vi "initialise__.vi"(8 "error in (no error)":errorcluster, 11 "GenericTrajectory in":refnum<class "TrajectoryDL110413StraightLine.lvclass">) -> (0 "error out":errorcluster, 3 "GenericTrajectory out":refnum<class "TrajectoryDL110413StraightLine.lvclass">)   [LabVIEW 2010]
uses:
  <vilib>/Analysis/NI_AALBase.lvlib
  <vilib>/Analysis/1siggen.llb/Ramp Pattern by Samples.vi
  TrajectoryDL110413StraightLine.lvclass
  common/enumerations/functional_global_action_enum.ctl
  common/enumerations/x_y_z_enumeration.ctl
  common/classes/ImageCollection/ImageCollection/ImageCollection.lvclass
  common/classes/Image/Image/Image.lvclass
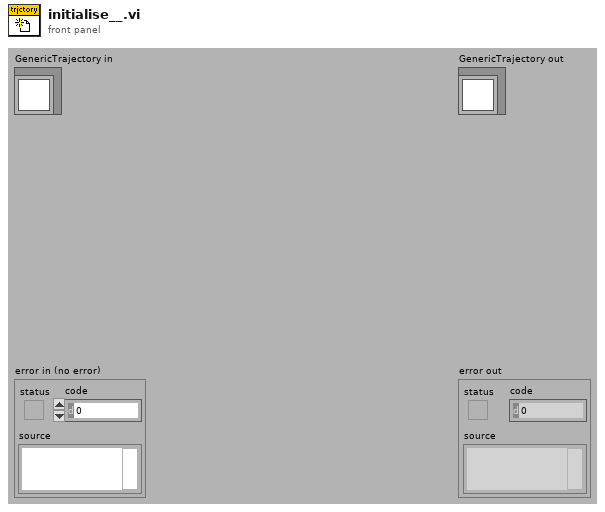
[diagram p1: front panel]
types:
  T1 = typedef "x_y_z_enumeration.ctl" = enum16{"x", "y", "z"}
  T2 = typedef "functional_global_action_enum.ctl" = enum16{"get", "set", "reset"}
  T3 = cluster{"[0]":void, "[1]":void, "[2]":void, "[3]":void}
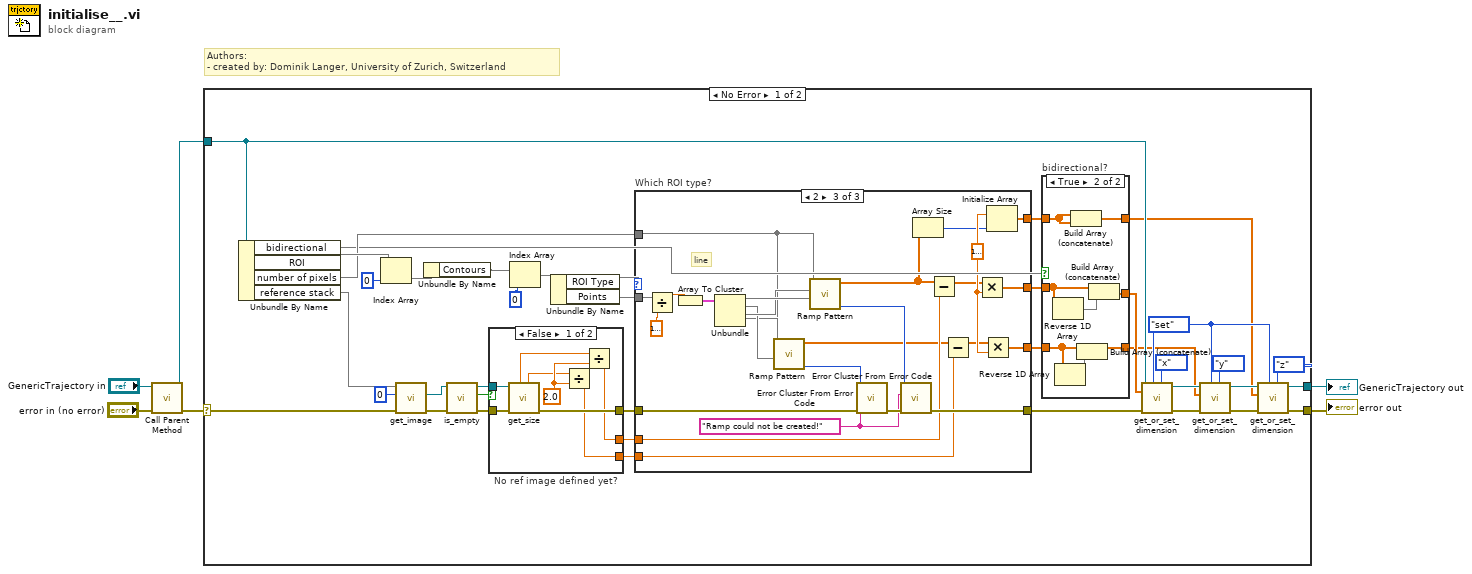
[diagram p0: block diagram]
diagram:
  # "Authors: \n- created by: Dominik Langer, University of Zurich, Switzerland"
  n1 = call-parent "Call Parent Method"("error in (no error)"="error in (no error)", "GenericTrajectory in"="GenericTrajectory in") -> ("error out"=w4:errorcluster, "GenericTrajectory out"=w3:refnum<class "TrajectoryDL110413StraightLine.lvclass">)  [unwired: 8 in]
  n2 = case shown="No Error" w4 {
    selector: w4 -> [w22 w94]
    tunnel: w3 -> [w36 w95]
    tunnel: [w29 w95] -> w2
    tunnel: [w27 w94] -> w1
    frame No Error {
      w26 = functional_global_action_enum."set" ("action")
      n3 = Unbundle By Name(w36) -> ("bidirectional"=w9, "ROI"=w45, "number of pixels"=w37, "reference stack"=w24)
      n4 = Index Array(array=w45, index=0) -> (element=w43)
      n5 = call-dynamic "get_image.vi"("error in (no error)"=w22, "index"=0, "ImageCollection in"=w24) -> ("error out"=w18:errorcluster, "Image.lvclass"=w16:refnum<class "Image.lvclass">)  [unwired: 6 in, 1 out]
      n6 = Unbundle By Name(w43) -> ("Contours"=w41)
      n7 = call-dynamic "is_empty.vi"("error in (no error)"=w18, "Image in"=w16) -> ("error out"=w17:errorcluster, "emtpy?"=w14:bool, "Image out"=w15:refnum<class "Image.lvclass">)  [unwired: 7 in]
      n8 = case "No ref image defined yet?" shown="False" w14 {
        tunnel: [w64 w65] -> w21
        tunnel: [w61 _] -> w20
        tunnel: [w59 _] -> w19
        tunnel: w17 -> [w58 w65]
        tunnel: w15 -> [w57 _]
        frame False {
          w63 = 2.0 ("y")
          n9 = call-dynamic "get_size.vi"("error in (no error)"=w58, "Image in"=w57) -> ("error out"=w64:errorcluster, "physical size y"=w60:dbl, "physical size x"=w62:dbl)  [unwired: 2 in, 5 out]
          n10 = Divide(x=w60, y=w63) -> (x/y=w59:dbl)
          n11 = Divide(x=w62, y=w63) -> (x/y=w61:dbl)
        }
        frame True {
        }
      }
      n12 = Index Array(array=w41, index=0) -> (element=w40)
      n13 = Unbundle By Name(w40) -> ("ROI Type"=w39, "Points"=w38)
      n14 = case "Which ROI type?" shown="2" w39 {
        tunnel: w38 -> [_ _ w91]
        tunnel: w37 -> [_ _ w68]
        tunnel: w21 -> [w66 w67 w84]
        tunnel: [w66 w67 w81] -> w34
        tunnel: [_ _ w75] -> w13
        tunnel: [_ _ w80] -> w10
        tunnel: [_ _ w77] -> w8
        tunnel: w20 -> [_ _ w74]
        tunnel: w19 -> [_ _ w71]
        frame Default {
        }
        frame 1 {
          # "single points..."
        }
        frame 2 {
          w76 = "Ramp could not be created!" ("error message (\"\")")
          w79 = dbl[unit] 1e-06 ("y")
          # "line"
          n15 = Divide(x=w91, y=dbl[unit] 1e-06) -> (x/y=w90:dbl)
          n16 = Array To Cluster(array=w90) -> (cluster=w93:T3)
          n17 = Unbundle(w93) -> ("[0]"=w89, "[1]"=w87, "[2]"=w88, "[3]"=w86)
          n18 = call-poly <vilib>:"Ramp Pattern.vi"("start"=w87, "end"=w86, "samples"=w68) -> ("error"=w85:i32, "Ramp Pattern"=w70:dbl[])  [unwired: 7 in]
          n19 = call-poly <vilib>:"Ramp Pattern.vi"("start"=w89, "end"=w88, "samples"=w68) -> ("error"=w83:i32, "Ramp Pattern"=w73:dbl[])  [unwired: 7 in]
          n20 = call <vilib>:"Error Cluster From Error Code.vi"("error in (no error)"=w84, "error message (\"\")"=w76, "error code (0)"=w85) -> ("error out"=w82:errorcluster)  [unwired: 6 in]
          n21 = call <vilib>:"Error Cluster From Error Code.vi"("error in (no error)"=w82, "error message (\"\")"=w76, "error code (0)"=w83) -> ("error out"=w81:errorcluster)  [unwired: 6 in]
          n22 = Array Size(array=w73) -> (size(s)=w78:i32)
          n23 = Subtract(x=w73, y=w74) -> (x-y=w72:dbl[])
          n24 = Subtract(x=w70, y=w71) -> (x-y=w69:dbl[])
          n25 = Multiply(x=w72, y=w79) -> (x*y=w75:dbl[unit][])
          n26 = Multiply(x=w69, y=w79) -> (x*y=w80:dbl[unit][])
          n27 = Initialize Array(w79, w78) -> (w77:dbl[unit][])
        }
      }
      n28 = case "bidirectional?" shown="True" w9 {
        tunnel: w13 -> [w47 w56]
        tunnel: [w47 w54] -> w12
        tunnel: [w48 w52] -> w11
        tunnel: w10 -> [w48 w51]
        tunnel: w8 -> [w46 w50]
        tunnel: [w46 w49] -> w7
        frame False {
        }
        frame True {
          n29 = Reverse 1D Array(array=w56) -> (reversed array=w55:dbl[unit][])
          n30 = Reverse 1D Array(array=w51) -> (reversed array=w53:dbl[unit][])
          n31 = Build Array (concatenate)(w50, w50) -> (w49:dbl[unit][])
          n32 = Build Array (concatenate)(w51, w53) -> (w52:dbl[unit][])
          n33 = Build Array (concatenate)(w56, w55) -> (w54:dbl[unit][])
        }
      }
      n34 = call-dynamic "get_or_set_dimension.vi"("dimension"=x_y_z_enumeration."x", "action"=w26, "error in (no error)"=w34, "pixel values in (single dimension)"=w12, "GenericTrajectory in"=w36) -> ("error out"=w35:errorcluster, "GenericTrajectory out"=w33:refnum<class "TrajectoryDL110413StraightLine.lvclass">)  [unwired: 4 in, 1 out]
      n35 = call-dynamic "get_or_set_dimension.vi"("dimension"=x_y_z_enumeration."y", "action"=w26, "error in (no error)"=w35, "pixel values in (single dimension)"=w11, "GenericTrajectory in"=w33) -> ("error out"=w28:errorcluster, "GenericTrajectory out"=w30:refnum<class "TrajectoryDL110413StraightLine.lvclass">)  [unwired: 4 in, 1 out]
      n36 = call-dynamic "get_or_set_dimension.vi"("dimension"=x_y_z_enumeration."z", "action"=w26, "error in (no error)"=w28, "pixel values in (single dimension)"=w7, "GenericTrajectory in"=w30) -> ("error out"=w27:errorcluster, "GenericTrajectory out"=w29:refnum<class "TrajectoryDL110413StraightLine.lvclass">)  [unwired: 4 in, 1 out]
    }
    frame Error {
    }
  }
  "error out" <- w1
  "GenericTrajectory out" <- w2
